vi "Center of mass 1d.vi"(11 "Data in":u8[](array[numeric])) -> (2 "Average value":dbl, 3 "Center of mass offset":dbl)   [LabVIEW 2013]
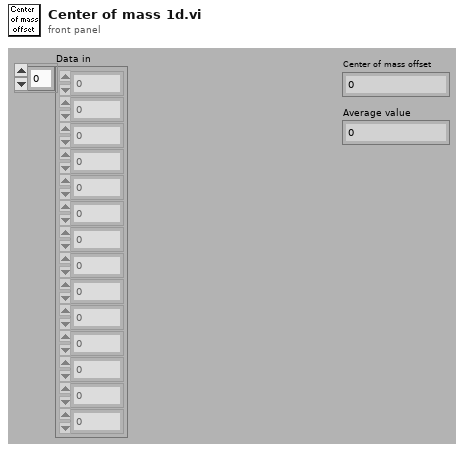
[diagram p1: front panel]
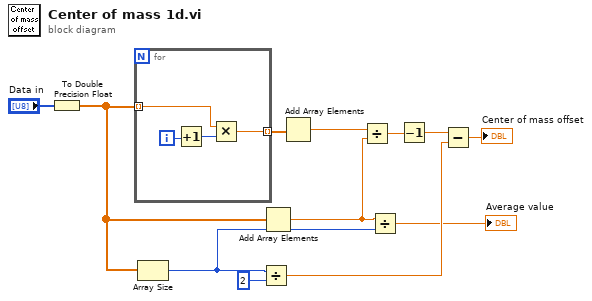
[diagram p0: block diagram]
diagram:
  n1 = To Double Precision Float(number="Data in") -> (double precision float=w6:dbl[])
  n2 = for {
    tunnel: w6 -> [w16] mode=indexing
    tunnel: [w15] -> w12 mode=indexing
    i -> [w14]
    n3 = Increment(x=w14) -> (x+1=w13:i32)
    n4 = Multiply(x=w16, y=w13) -> (x*y=w15:dbl)
  }
  n5 = Array Size(array=w6) -> (size(s)=w2:i32)
  n6 = Divide(x=w2, y=2) -> (x/y=w9:dbl)
  n7 = Add Array Elements(numeric array=w6) -> (sum=w3:dbl)
  n8 = Add Array Elements(numeric array=w12) -> (sum=w11:dbl)
  n9 = Divide(x=w11, y=w3) -> (x/y=w4:dbl)
  n10 = Divide(x=w3, y=w2) -> (x/y=→"Average value":dbl)
  n11 = Decrement(x=w4) -> (x-1=w5:dbl)
  n12 = Subtract(x=w5, y=w9) -> (x-y=→"Center of mass offset":dbl)
